vi "Record Call.vi"(8 "error in (no error)":errorcluster, 10 "This VI":refnum<vi>, 11 "Mock In":refnum<class "Responsive Mock.lvclass">) -> (0 "error out":errorcluster, 3 "Mock Out":refnum<class "Responsive Mock.lvclass">)   [LabVIEW 2020, in "Responsive Mock.lvclass"]
uses:
  Responsive Mock.lvclass
  Responsive Mock.lvclass/Responsive Mock.ctl
  Core/Expectation/Expectation.lvclass
  VI Server VI Call/VI Server VI Call.lvclass
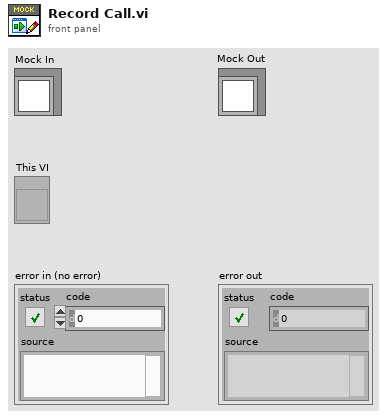
[diagram p1: front panel]
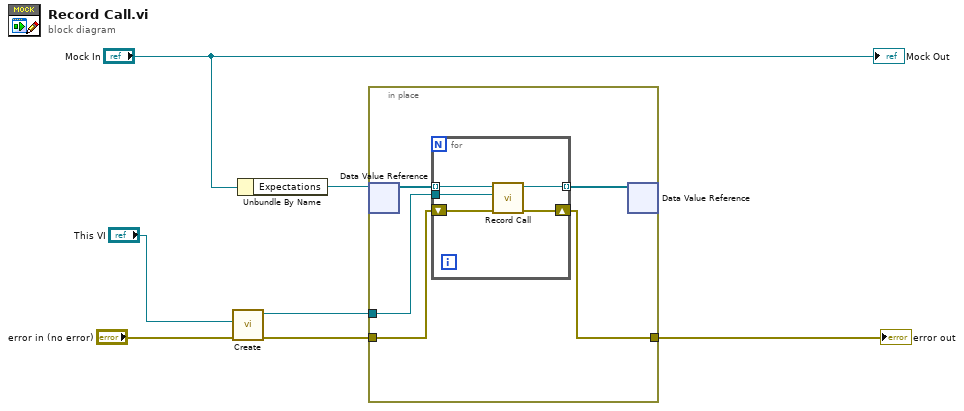
[diagram p0: block diagram]
diagram:
  n1 = call "Create.vi"("error in (no error)"="error in (no error)", "VI"="This VI") -> ("error out"=w3:errorcluster, "Call Out"=w1:refnum<class "VI Server VI Call.lvclass">)  [unwired: 8 in]
  n2 = Unbundle By Name("Mock In") -> ("Expectations"=w7:refnum<data-value>)
  n3 = in-place {
    in-place-border: [w12] -> w5
    in-place-border: w3 -> [w11]
    in-place-border: w1 -> [w8]
    n4 = in-place-dvr #1(w7) -> (w10:refnum<class "Expectation.lvclass">[])  [unwired: 1 out]
    n5 = for {
      tunnel: w10 -> [w17] mode=indexing
      tunnel: [w16] -> w9 mode=indexing
      shift-right: [w15] -> w12
      shift-left: w11 -> [w14]
      tunnel: w8 -> [w13]
      n6 = call-dynamic "Record Call.vi"("error in (no error)"=w14, "VI Call"=w13, "Expectation in"=w17) -> ("error out"=w15:errorcluster, "Expectation out"=w16:refnum<class "Expectation.lvclass">)  [unwired: 7 in]
    }
    n7 = in-place-dvr #1(w9) -> ()  [unwired: 2 out]
  }
  "error out" <- w5
  "Mock Out" <- "Mock In"
